vi "Init Events.vi"(8 "error in (no error)":errorcluster, 11 "ChannelService in":refnum<class "ChannelService.lvclass">) -> (0 "error out":errorcluster, 3 "ChannelService out":refnum<class "ChannelService.lvclass">)   [LabVIEW 2020, in "Vecto.lvlib" / "ChannelService.lvclass"]
uses:
  ChannelService.lvclass
  New Group Data.ctl
  Group Config/Group Config.lvclass
  <vilib>/IlluminatedG/IG Promises/Promises/Promise/Promise.lvclass
  Incoming Events.ctl
  Lookup Channel Data.ctl
  ChannelService.lvclass/ChannelService.ctl
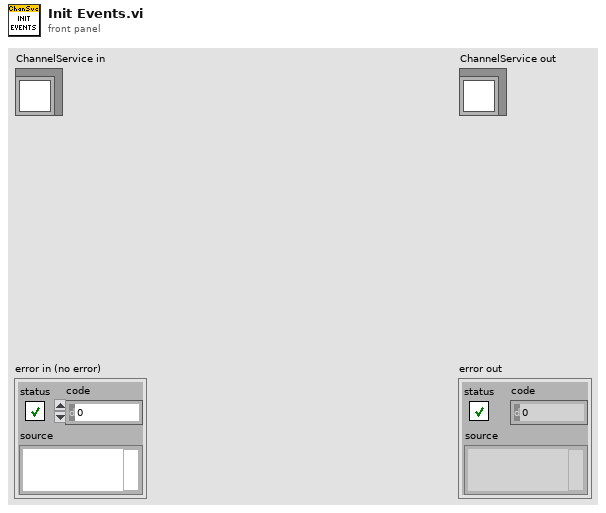
[diagram p1: front panel]
types:
  T1 = typedef "Vecto.lvlib/ChannelService.lvclass/Lookup Channel Data.ctl" = cluster{"Channel Name":string, "Promise":refnum<class "Promise.lvclass">}
  T2 = typedef "Vecto.lvlib/ChannelService.lvclass/Incoming Events.ctl" = cluster{"New Group":refnum<user-event>, "Close":refnum<user-event>, "Lookup Channel":refnum<user-event>}
  T3 = typedef "Vecto.lvlib/ChannelService.lvclass/New Group Data.ctl" = cluster{"Group Config":refnum<class "Group Config.lvclass">, "Promise":refnum<class "Promise.lvclass">}
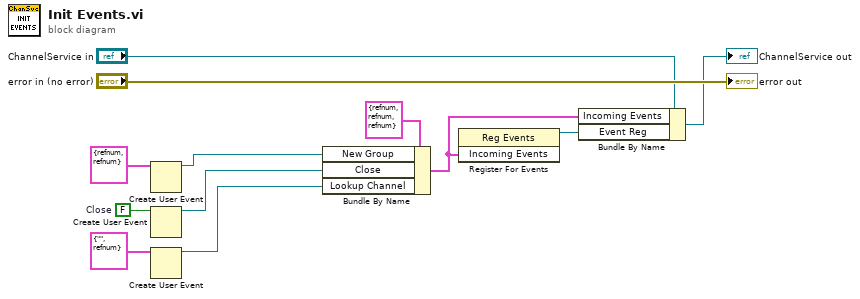
[diagram p0: block diagram]
diagram:
  w4 = FALSE  # Close
  n1 = Create User Event(user event datatype=T3 {"Group Config"=refnum, "Promise"=refnum} ("New Group Data")) -> (user event=w9:refnum<user-event>)  [unwired: 1 in, 1 out]
  n2 = Create User Event(user event datatype=w4) -> (user event=w3:refnum<user-event>)  [unwired: 1 in, 1 out]
  n3 = Create User Event(user event datatype=T1 {"Channel Name"="", "Promise"=refnum} ("Lookup Channel Data")) -> (user event=w1:refnum<user-event>)  [unwired: 1 in, 1 out]
  n4 = Bundle By Name(cluster=T2 {"New Group"=refnum, "Close"=refnum, "Lookup Channel"=refnum} ("Incoming Events"), "New Group"=w9, "Close"=w3, "Lookup Channel"=w1) -> (w6:T2)
  n5 = register-events(w6) -> (reference out=w7:refnum<event-registration>)  [unwired: 2 in, 1 out]
  n6 = Bundle By Name(cluster="ChannelService in", "Incoming Events"=w6, "Event Reg"=w7) -> (→"ChannelService out":refnum<class "ChannelService.lvclass">)
  "error out" <- "error in (no error)"
